vi "process.vi"() -> ()   [LabVIEW 2012]
uses:
  <vilib>/vision/Image Controls.llb/IMAQ Image.ctl
  <vilib>/vision/NI_Vision_Development_Module.lvlib
panel:
  out "targetCount":i32
  in  "Save":bool
  out "imageCount":i32
  in  "Existing Target":bool
  out "Identified Targets":T2(array[cluster]) {"Orientation" items=["North", "North-East", "East", "South-East", "South", "South-West", "West", "North-West"]; "Cluster"."Longitude" format="%#_10g"; "Cluster"."Latitude" format="%#_10g"}
  out "data":string
  out "state":i32
  in  "New Target Button":bool
  in  "currentImage":i32
  out "Image Out":T1(plugin-control)
  out "reloadImage":refnum<user-event>
  in  "prevbutton":bool
  in  "nextButton":bool
  in  "stop":bool
  out "Image Count":i32
  out "Available Images":i32[](array[numeric])
  # "of"
  # "of"
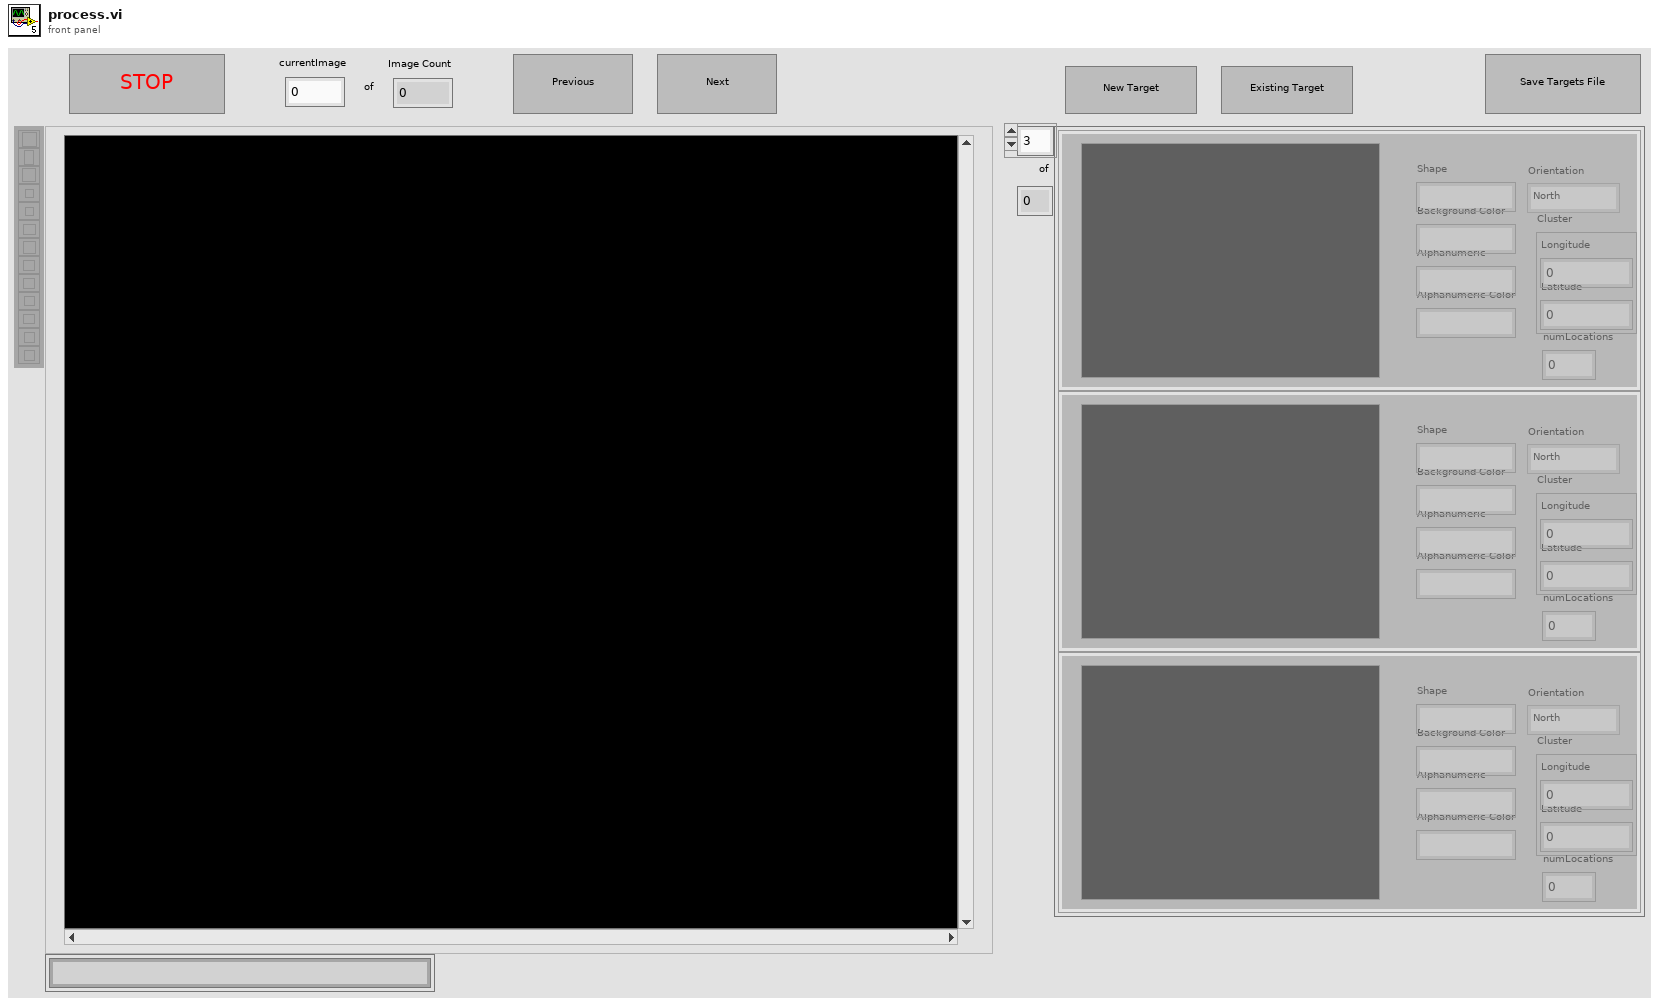
[diagram p1: front panel]
types:
  T1 = typedef "IMAQ Image.ctl" = refnum<image>
  T2 = cluster{"Image Out":T1, "Shape":string, "Background Color":string, "Alphanumeric":string, "Alphanumeric Color":string, "Cluster":cluster{"Longitude":dbl, "Latitude":dbl}, "Orientation":u16, "numLocations":i32}[]
  T3 = cluster{"Global Rectangle":i32[], "Contours":cluster{"Contour Type":u32, "ROI Type":u32, "Points":i32[]}[]}
  T4 = enum16{"open", "replace", "create", "open or create", "replace or create", "replace or create with confirmation"}
  T5 = cluster{"Shift":bool, "Ctrl":bool, "Alt":bool, "Cmd":bool, "Opt":bool}
  T6 = typedef "Image Type" = u32
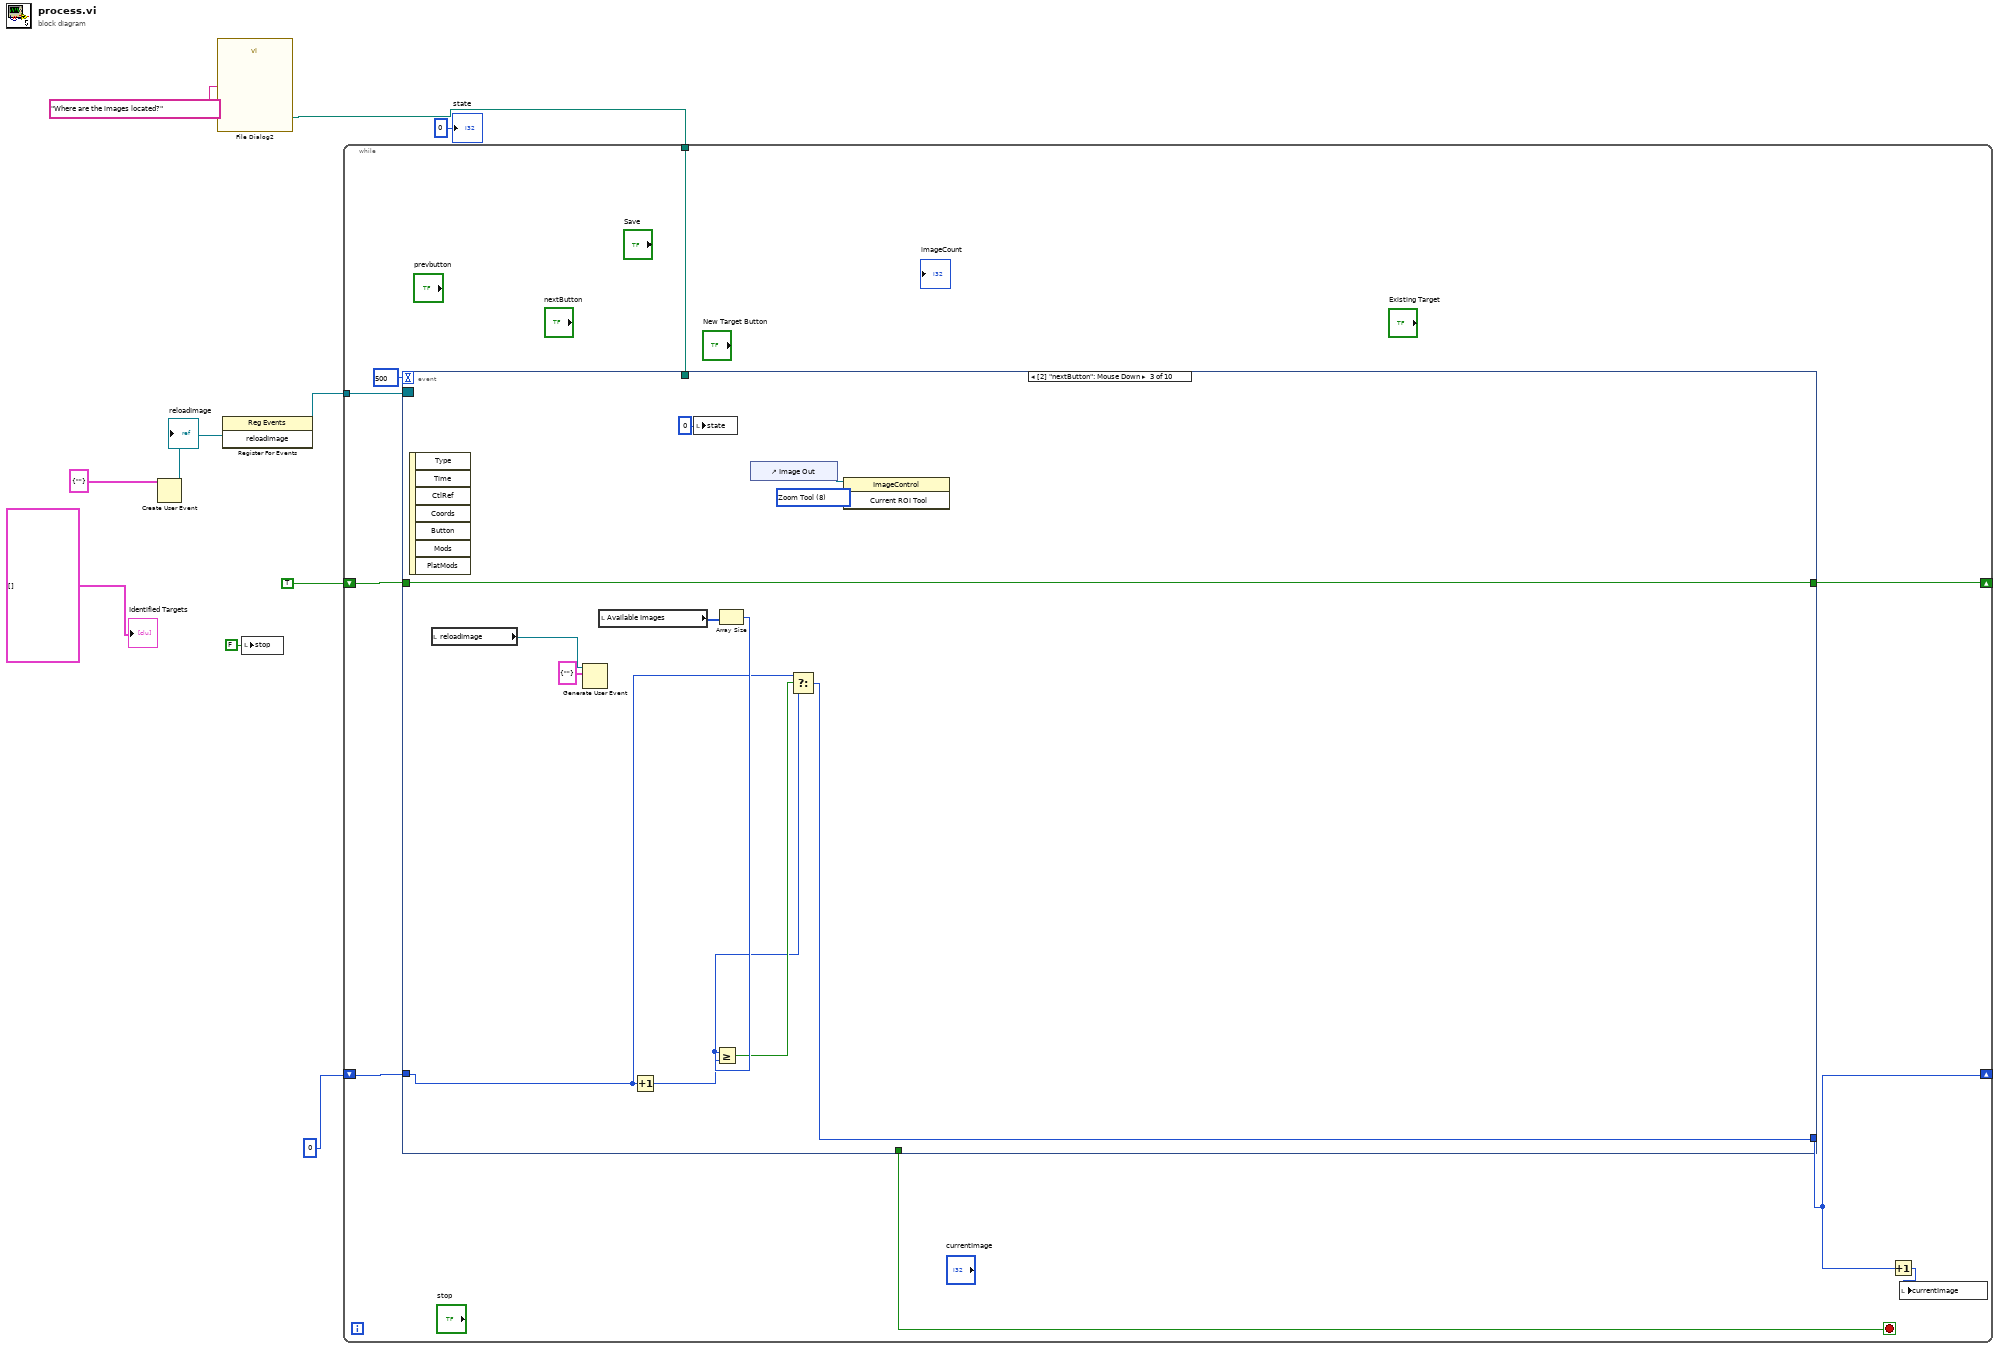
[diagram p0: block diagram]
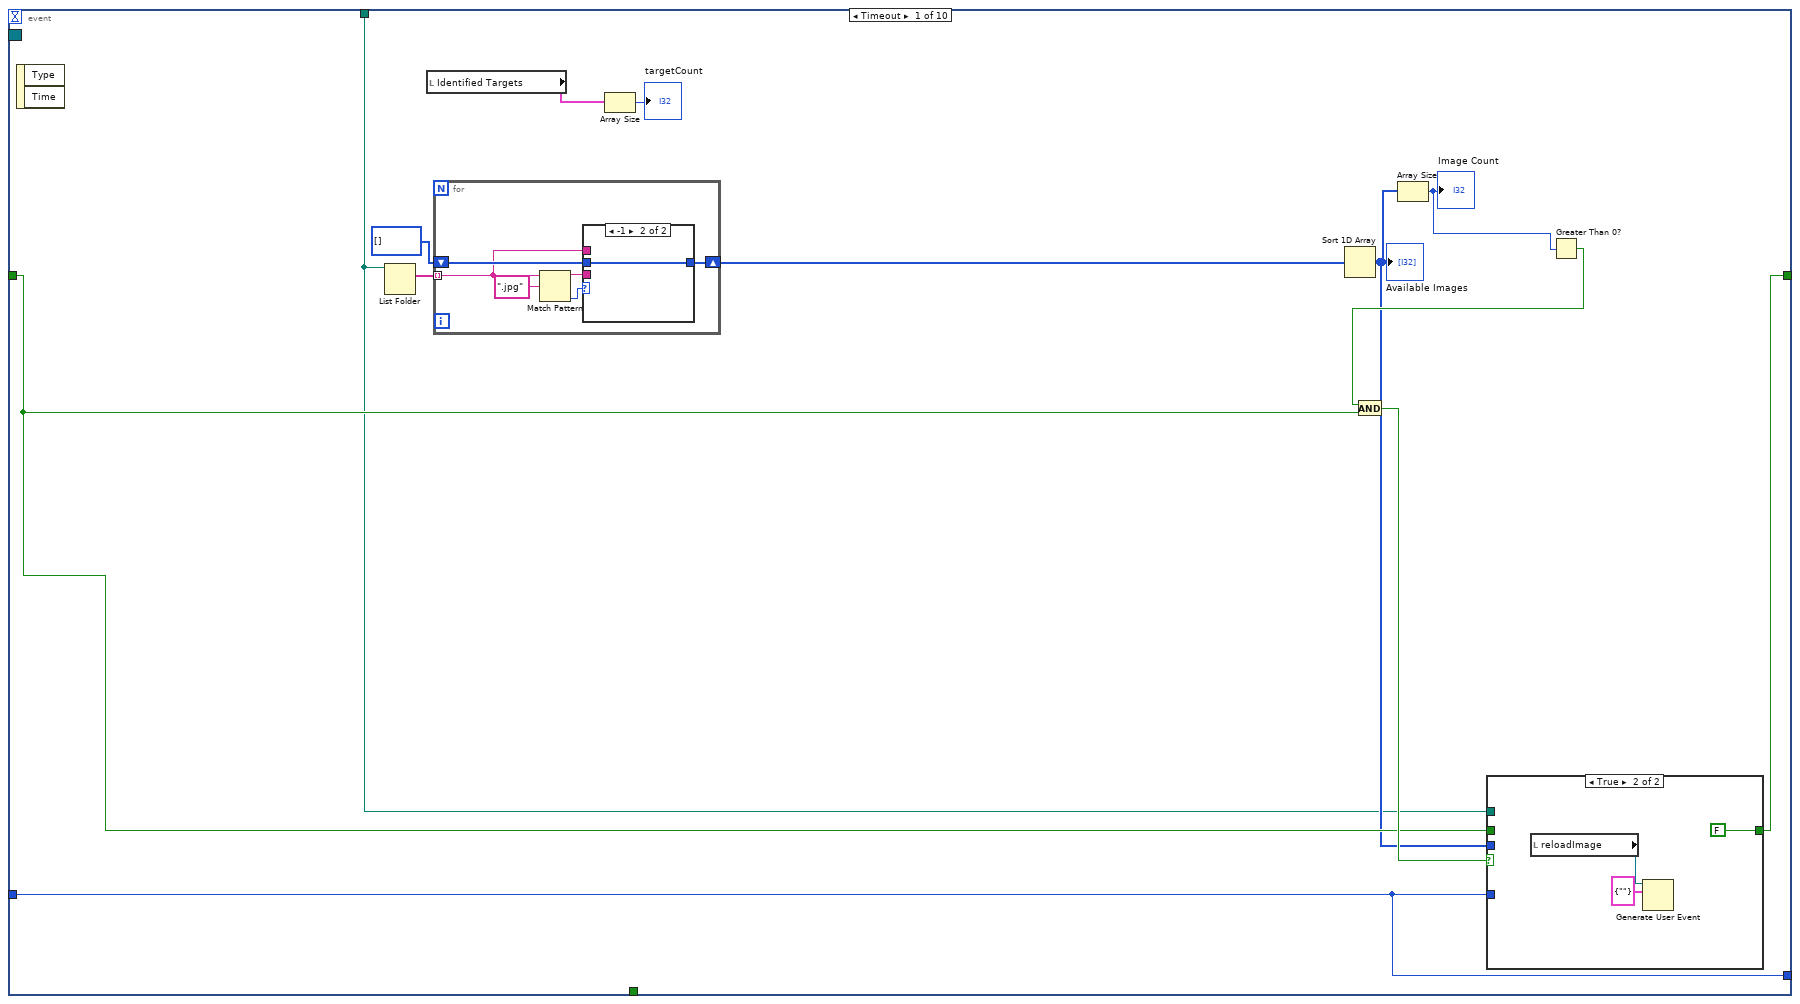
[diagram p2: hidden frame]
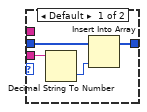
[diagram p4: hidden frame]
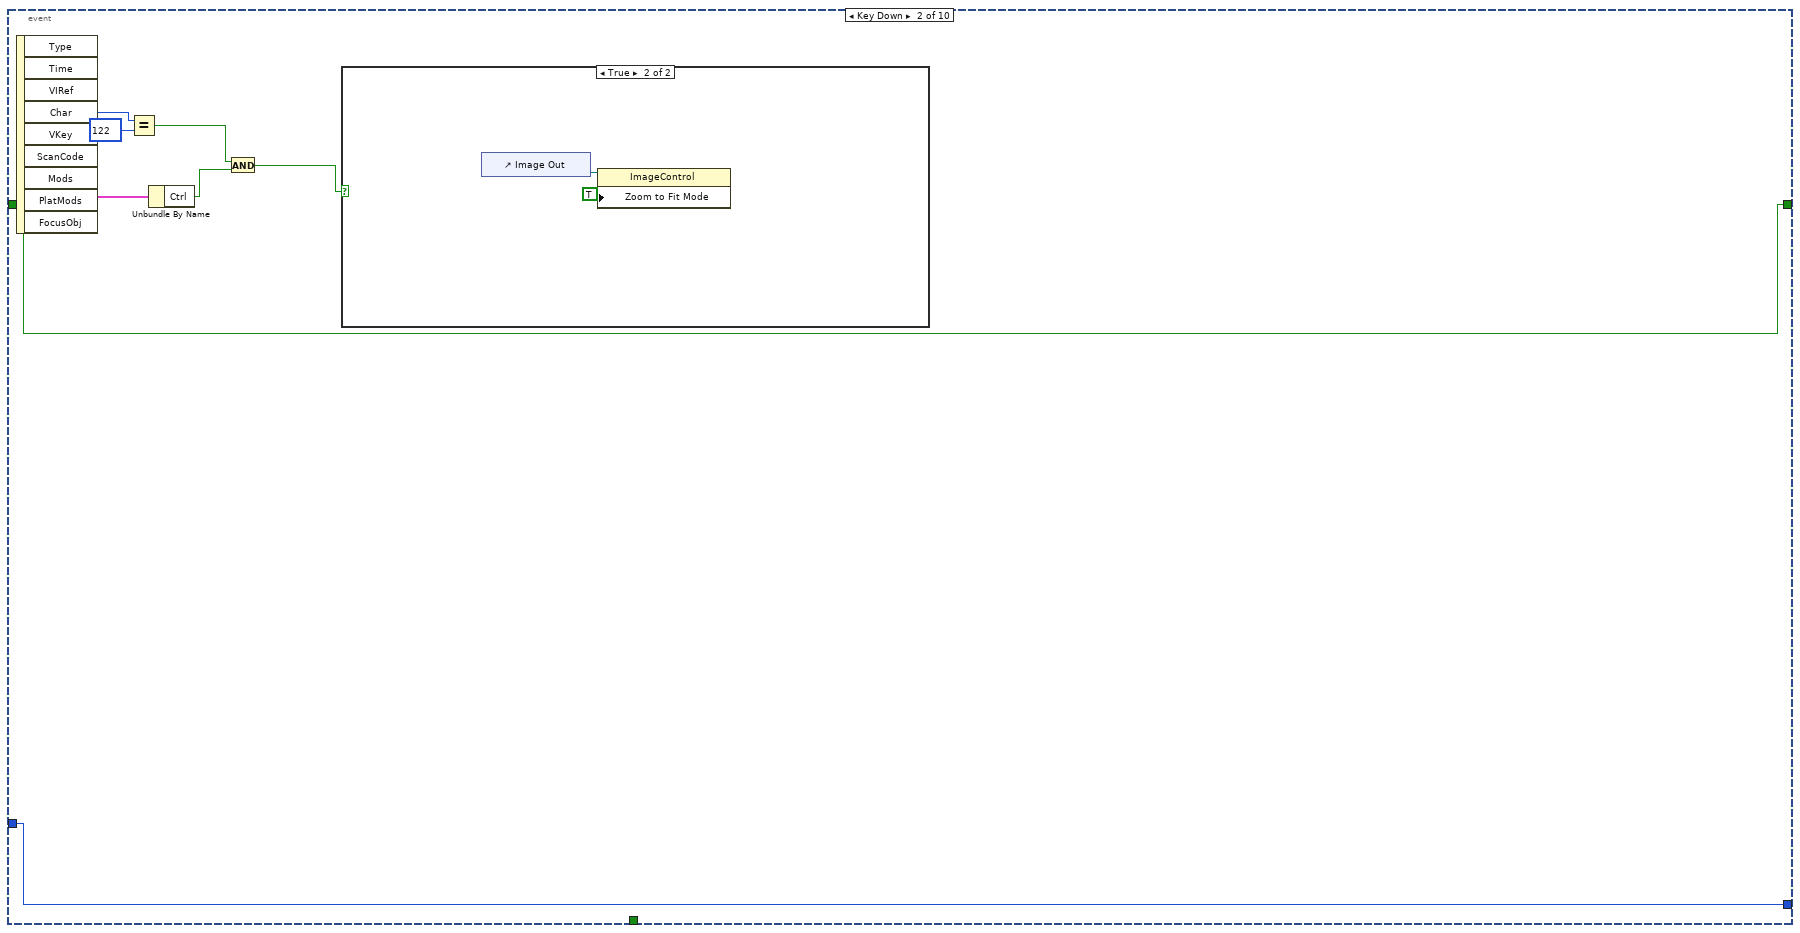
[diagram p5: hidden frame]
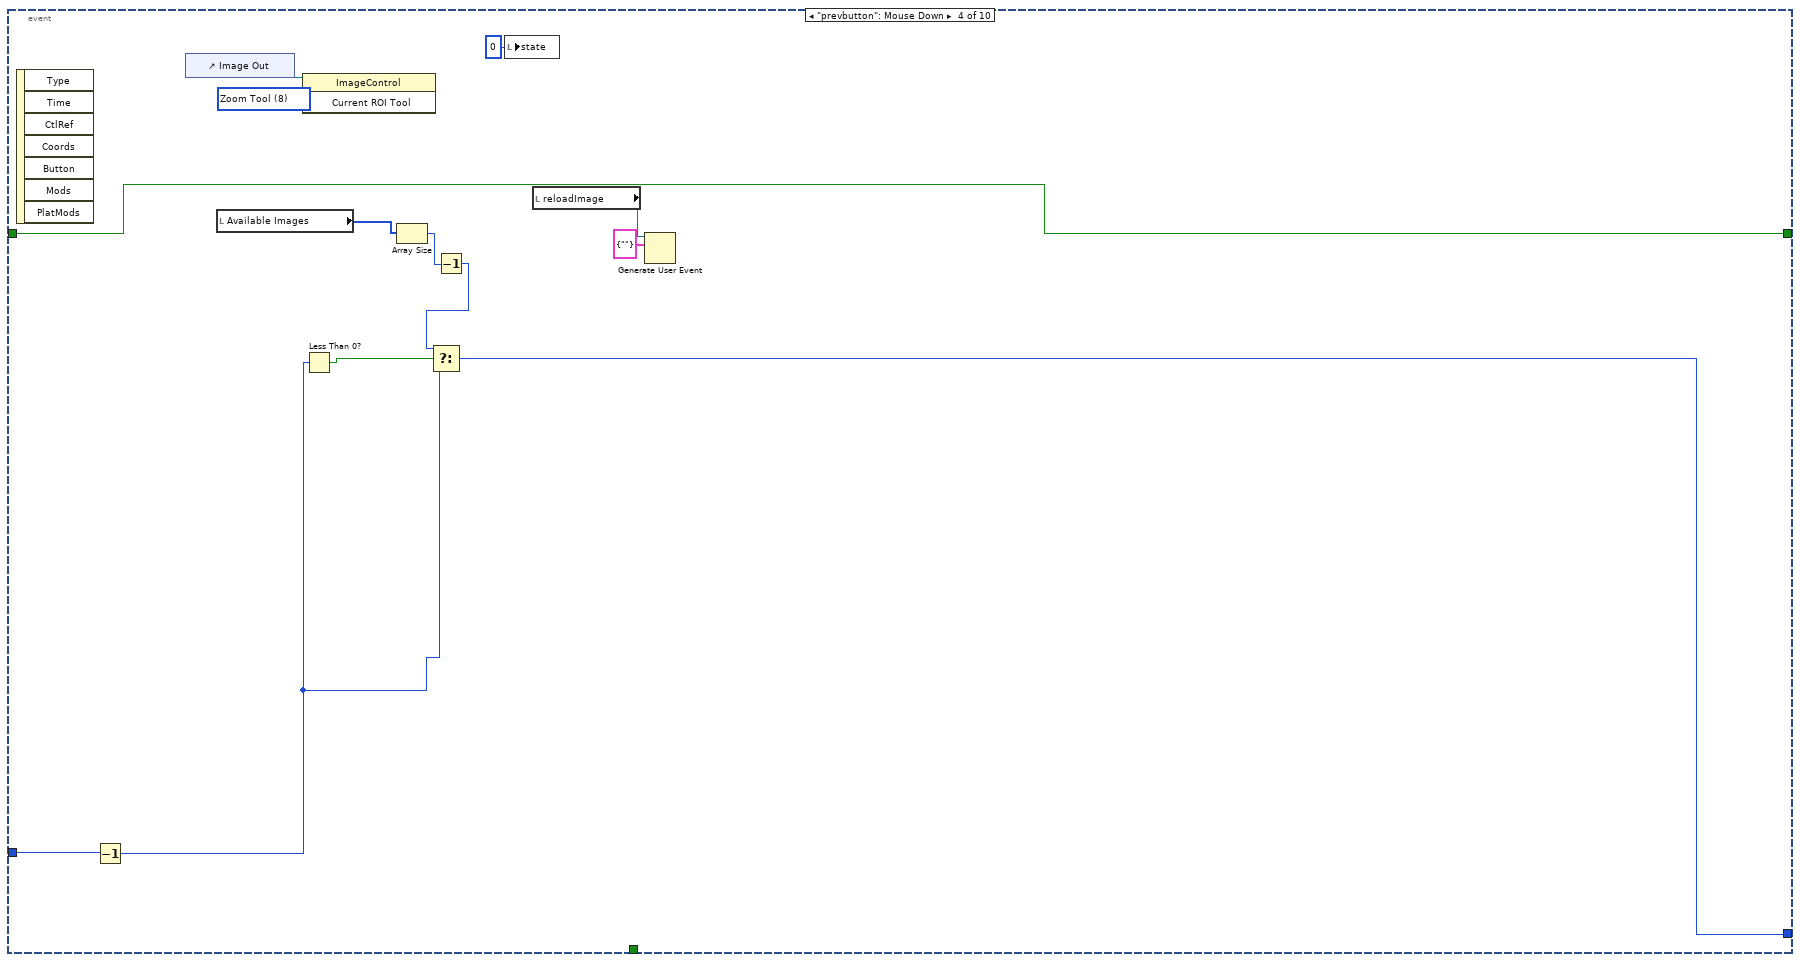
[diagram p7: hidden frame]
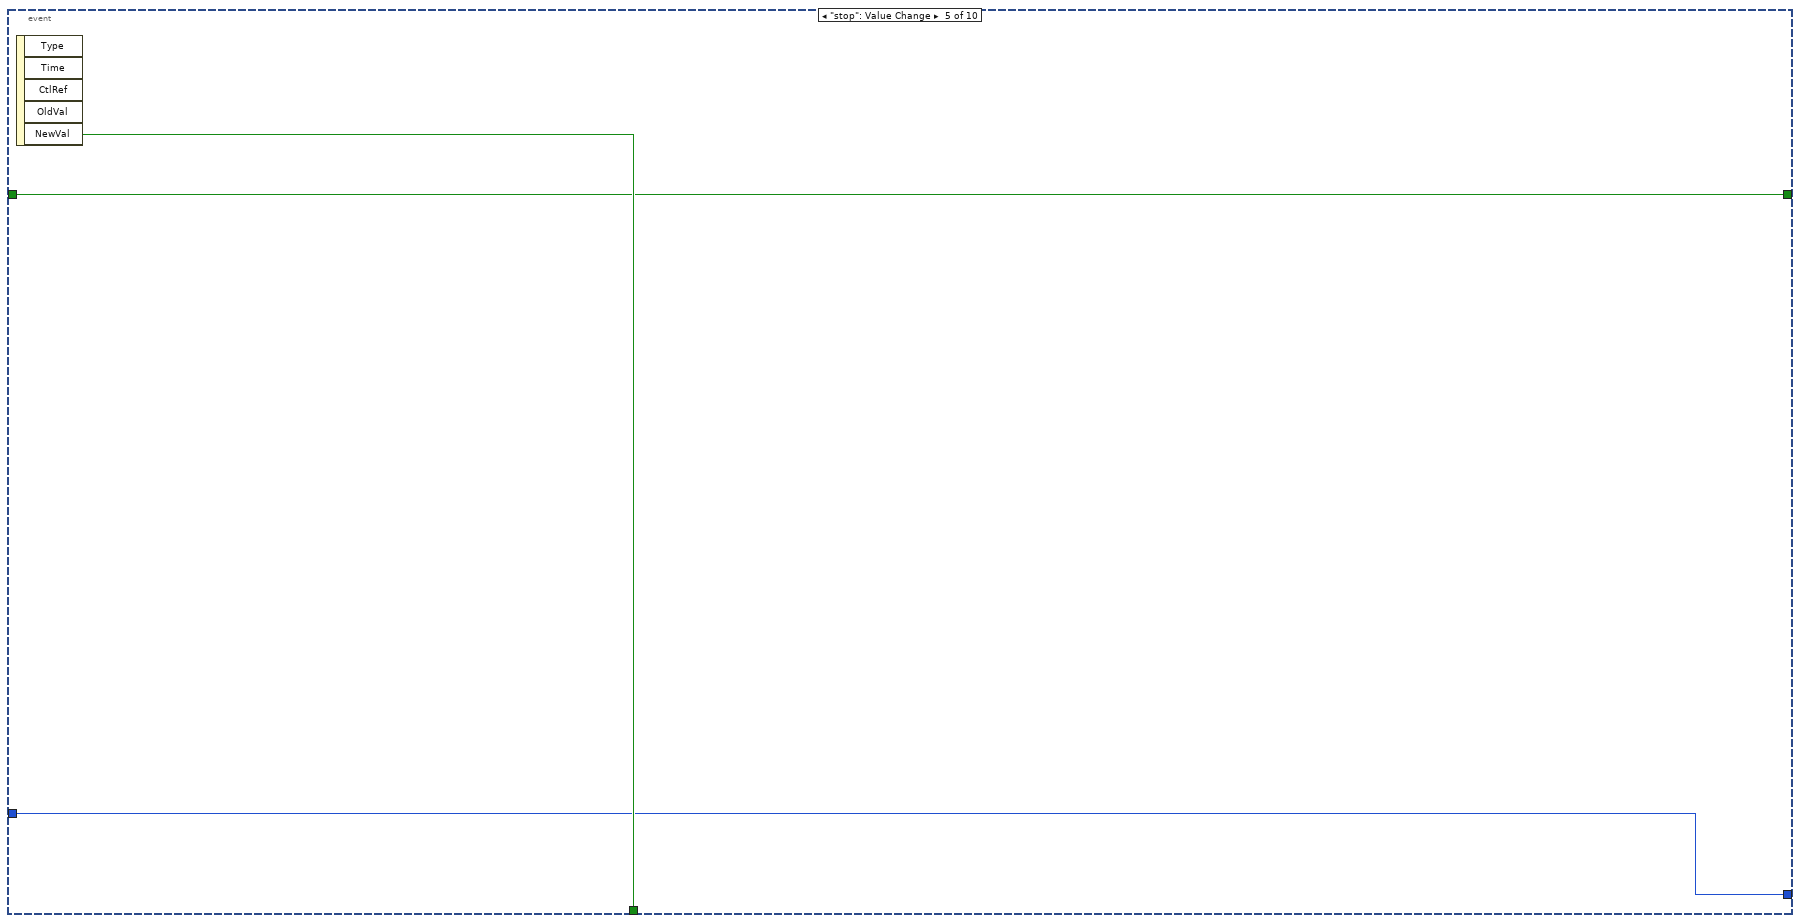
[diagram p8: hidden frame]
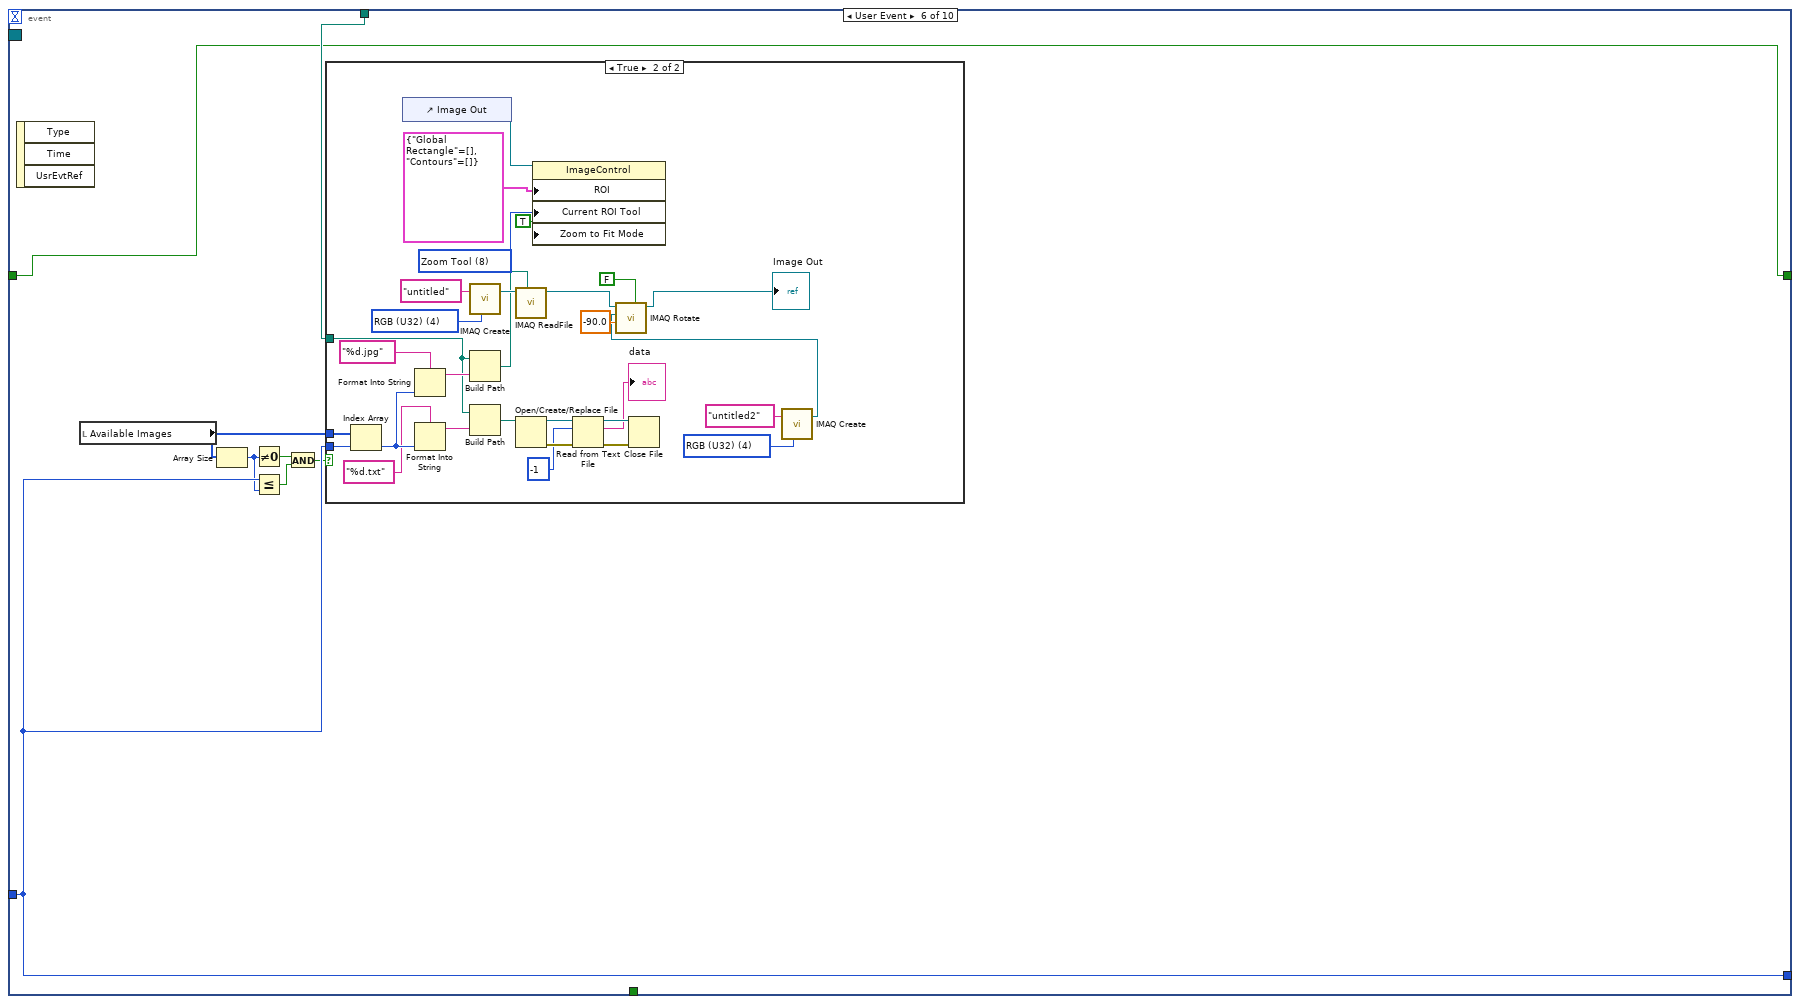
[diagram p9: hidden frame]
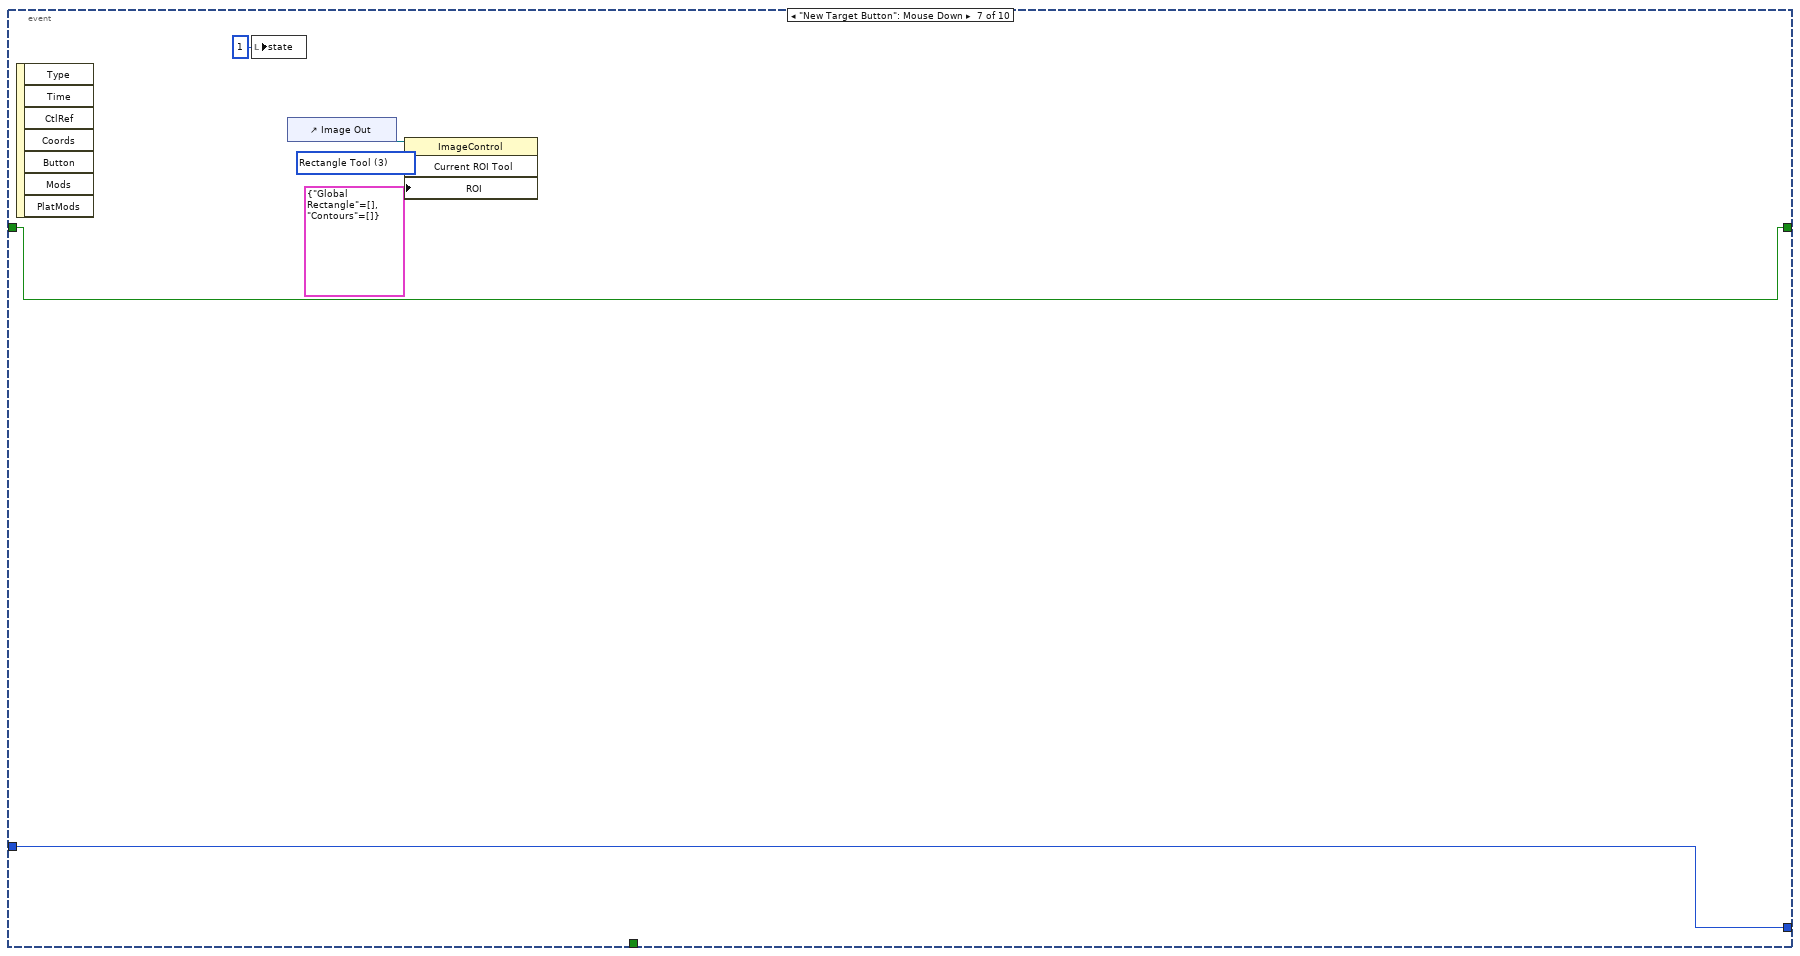
[diagram p11: hidden frame]
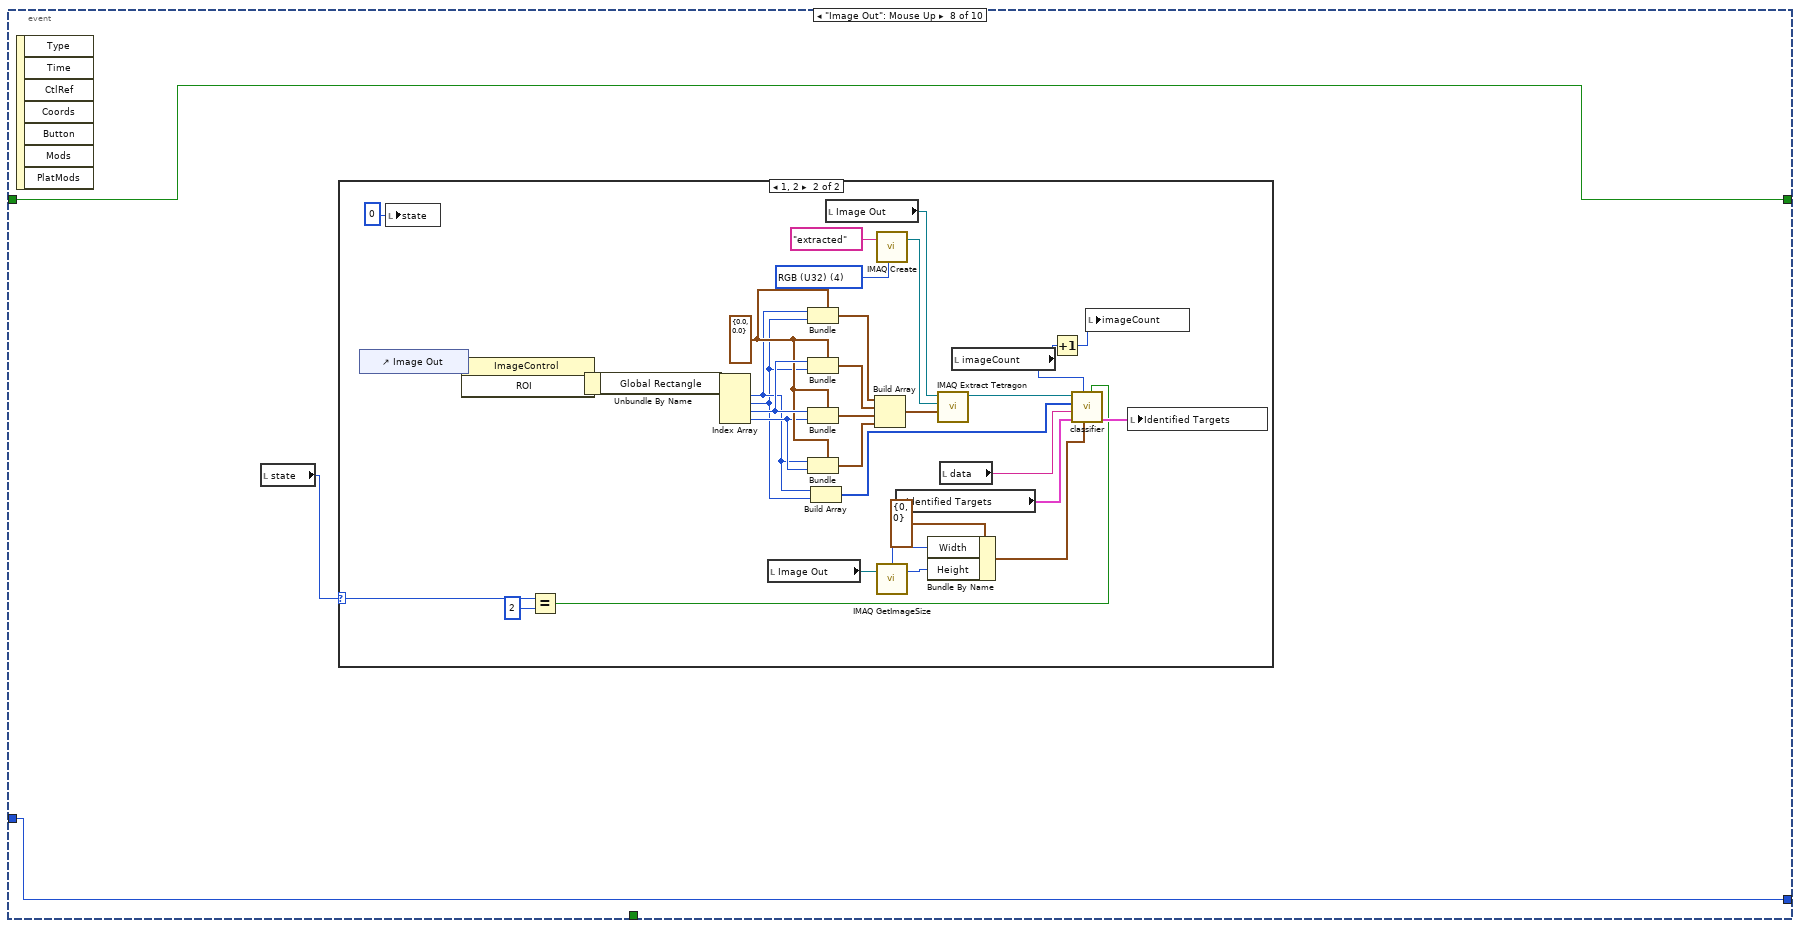
[diagram p12: hidden frame]
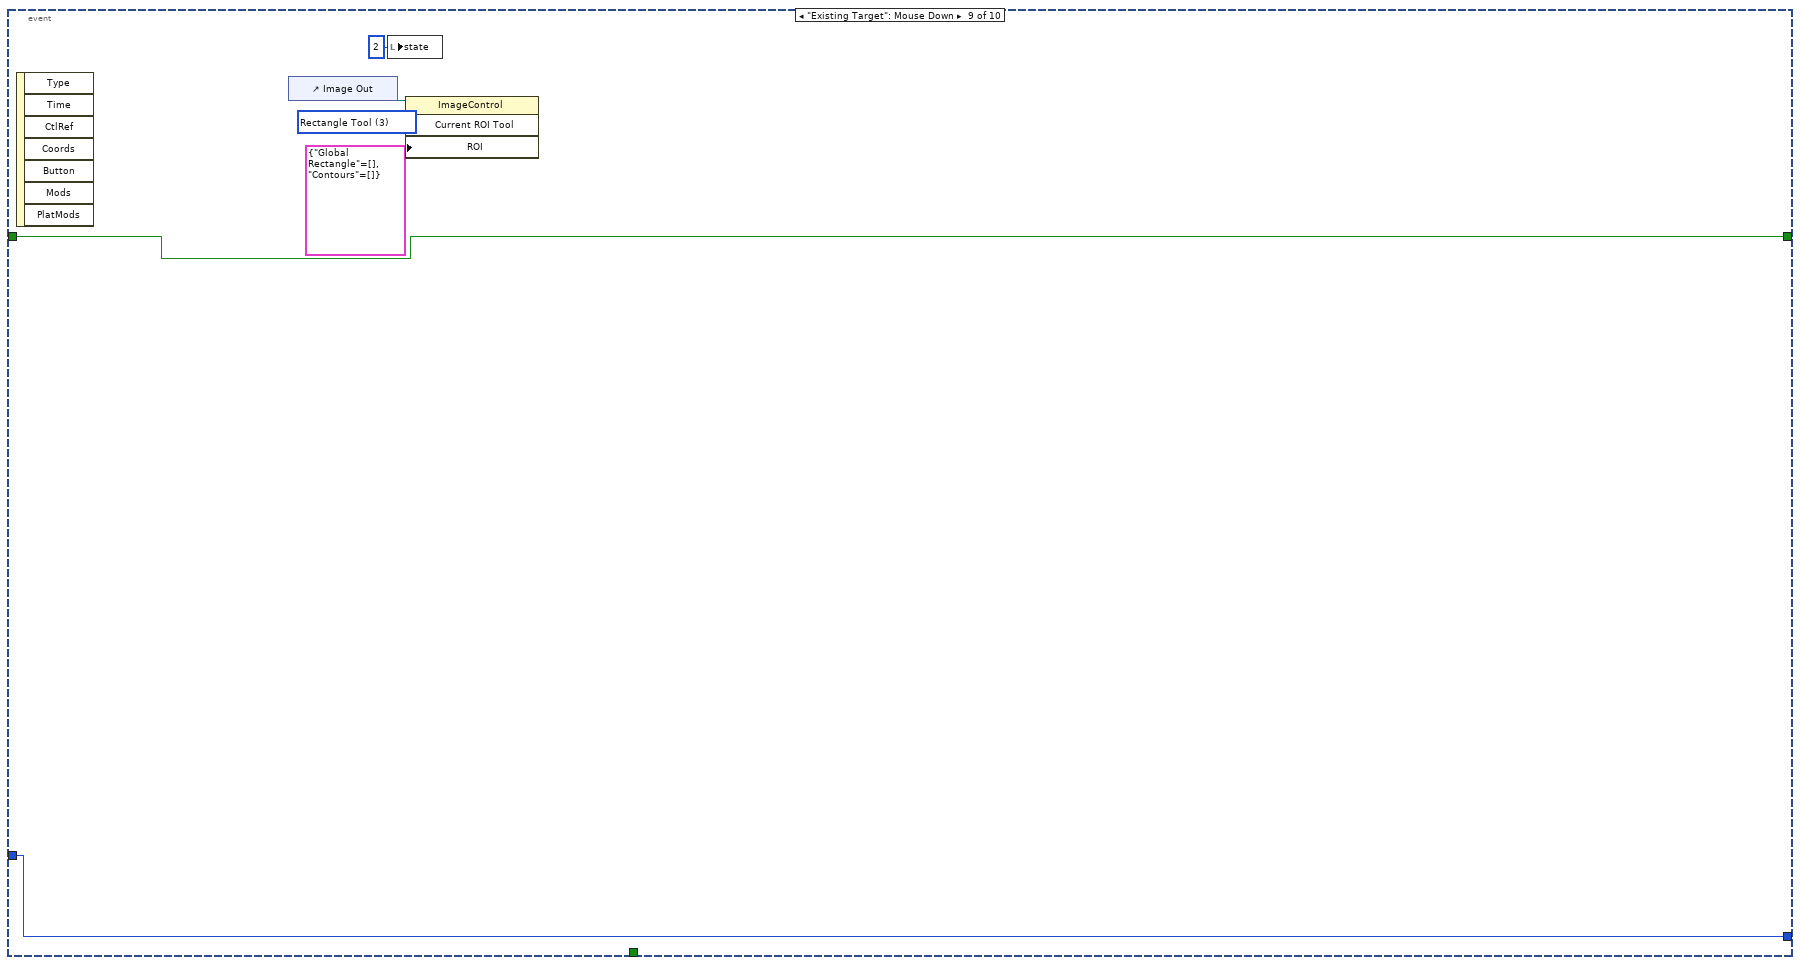
[diagram p14: hidden frame]
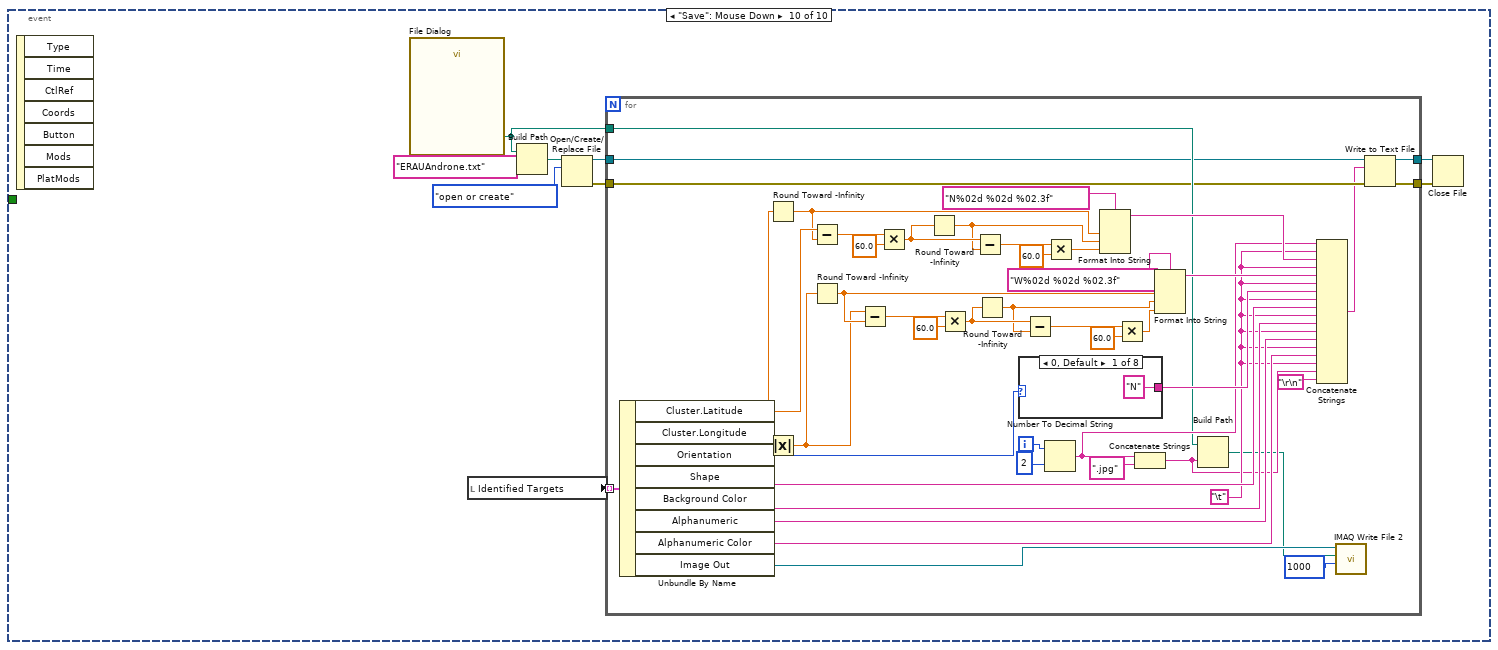
[diagram p15: hidden frame]
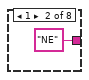
[diagram p16: hidden frame]
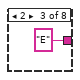
[diagram p17: hidden frame]
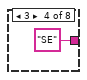
[diagram p18: hidden frame]
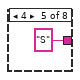
[diagram p19: hidden frame]
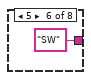
[diagram p20: hidden frame]
diagram:
  n1 = Create User Event(user event datatype=cluster{"stringy":string} {"stringy"=""} ("reloadImage")) -> (user event=w7:refnum<user-event>)  [unwired: 1 in, 1 out]
  "reloadImage" <- w7
  n2 = call "File Dialog2"("prompt"="Where are the images located?") -> ("selected path"=w3:path)  [unwired: 11 in, 3 out]
  n3 = register-events(w7) -> (reference out=w6:refnum<event-registration>)  [unwired: 2 in, 1 out]
  n4 = local write "stop"(FALSE ("stop")) -> ()
  n5 = while {
    shift-right: [w16] -> _
    shift-left: TRUE -> [w17]
    shift-right: [w14] -> _
    shift-left: 0 -> [w15]
    tunnel: w6 -> [w13]
    tunnel: w3 -> [w12]
    stop <- w18 stop-if-true
    n6 = event shown="[2] \"nextButton\": Mouse Down" {
      selector: w13 -> [_ _ _ _ _ _ _ _ _ _]
      dyn-events: _ -> [_ _ _ _ _ _ _ _ _ _]
      timeout: 500 -> [_ _ _ _ _ _ _ _ _ _]
      tunnel: [_ _ _ _ w85 _ _ _ _ _] -> w18
      tunnel: w17 -> [w25 w48 w69 w73 w83 w86 w126 w132 w166 _]
      tunnel: [w26 w48 w69 w73 w83 w86 w126 w132 w166 _] -> w16
      tunnel: w15 -> [w23 w49 w61 w82 w84 w92 w125 w131 w167 _]
      tunnel: [w23 w49 w62 w79 w84 w92 w125 w131 w167 _] -> w14
      tunnel: w12 -> [w22 _ _ _ _ w87 _ _ _ _]
      event Timeout {
        n7 = event-data() -> ()  [unwired: 1 in, 2 out]
        n8 = List Folder(path=w22) -> (filenames=w32:string[])  [unwired: 3 in, 3 out]
        n9 = local read "Identified Targets"() -> (w21:T2)
        n10 = for {
          tunnel: w32 -> [w39] mode=indexing
          shift-right: [w38] -> w30
          shift-left: i32[] [] -> [w40]
          n11 = Match Pattern(string=w39, regular expression=".jpg") -> (before substring=w37:string, offset past match=w41:i32)  [unwired: 1 in, 2 out]
          n12 = case shown="-1" w41 {
            tunnel: w40 -> [w46 w47]
            tunnel: w39 -> [_ _]
            tunnel: [w45 w47] -> w38
            tunnel: w37 -> [w44 _]
            frame Default {
              n13 = Decimal String To Number(string=w44) -> (number=w43:i32)  [unwired: 2 in, 1 out]
              n14 = Insert Into Array(array=w46, new element=w43) -> (w45:i32[])  [unwired: 1 in]
            }
            frame -1 {
            }
          }
        }
        n15 = Array Size(array=w21) -> (size(s)=→"targetCount":i32)
        n16 = Sort 1D Array(array=w30) -> (sorted array=w24:i32[])
        "Available Images" <- w24
        n17 = Array Size(array=w24) -> (size(s)=w28:i32)
        "Image Count" <- w28
        n18 = Greater Than 0?(x=w28) -> (x > 0?=w27:bool)
        n19 = And(x=w27, y=w25) -> (x .and. y?=w29:bool)
        n20 = case shown="True" w29 {
          tunnel: [w33 FALSE] -> w26
          tunnel: w25 -> [w33 _]
          tunnel: w24 -> [_ _]
          tunnel: w23 -> [_ _]
          tunnel: w22 -> [_ _]
          frame False {
          }
          frame True {
            n21 = local read "reloadImage"() -> (w35:refnum<user-event>)
            n22 = Generate User Event(user event=w35, event data cluster=cluster{"stringy":string} {"stringy"=""} ("event data")) -> ()  [unwired: 1 in, 2 out]
          }
        }
      }
      event Key Down {
        n23 = event-data() -> ("Char"=w54:i16, "PlatMods"=w55:T5)  [unwired: 1 in, 7 out]
        n24 = Equal?(x=w54, y=i16 122) -> (x = y?=w51:bool)
        n25 = Unbundle By Name(w55) -> ("Ctrl"=w52:bool)
        n26 = And(x=w51, y=w52) -> (x .and. y?=w50:bool)
        n27 = case shown="True" w50 {
          frame False {
          }
          frame True {
            n28 = control-ref of="Image Out"() -> (w57:refnum<vi>)
            n29 = property class="ImageControl"(reference=w57, "Zoom to Fit Mode"=TRUE) -> ()  [unwired: 1 in, 2 out]
          }
        }
      }
      event "nextButton": Mouse Down {
        w58 = u32 8 items=["Zoom Tool"=8, "Selection Tool"=0, "Pan Tool"=9, "Point Tool"=1, "Line Tool"=2, "Rectangle Tool"=3, "Rotated Rectangle Tool"=12, "Polyline Tool"=10, "Polygon Tool"=5, "Freehand Tool"=11, "Closed Freehand Tool"=6, "Ellipse Tool"=4, "Annulus Tool"=7] ("Current ROI Tool")
        n30 = event-data() -> ()  [unwired: 1 in, 7 out]
        n31 = local read "reloadImage"() -> (w68:refnum<user-event>)
        n32 = Generate User Event(user event=w68, event data cluster=cluster{"stringy":string} {"stringy"=""} ("event data")) -> ()  [unwired: 1 in, 2 out]
        n33 = local read "Available Images"() -> (w66:i32[])
        n34 = Increment(x=w61) -> (x+1=w63:i32)
        n35 = local write "state"(0 ("state")) -> ()
        n36 = Array Size(array=w66) -> (size(s)=w65:i32)
        n37 = Greater Or Equal?(x=w63, y=w65) -> (x >= y?=w64:bool)
        n38 = control-ref of="Image Out"() -> (w59:refnum<vi>)
        n39 = Select(t=w61, s=w64, f=w63) -> (s? t:f=w62:i32)
        n40 = property class="ImageControl"(reference=w59, "Current ROI Tool"=w58) -> ()  [unwired: 1 in, 2 out]
      }
      event "prevbutton": Mouse Down {
        w70 = u32 8 items=["Zoom Tool"=8, "Selection Tool"=0, "Pan Tool"=9, "Point Tool"=1, "Line Tool"=2, "Rectangle Tool"=3, "Rotated Rectangle Tool"=12, "Polyline Tool"=10, "Polygon Tool"=5, "Freehand Tool"=11, "Closed Freehand Tool"=6, "Ellipse Tool"=4, "Annulus Tool"=7] ("Current ROI Tool")
        n41 = event-data() -> ()  [unwired: 1 in, 7 out]
        n42 = Decrement(x=w82) -> (x-1=w80:i32)
        n43 = control-ref of="Image Out"() -> (w71:refnum<vi>)
        n44 = local read "Available Images"() -> (w78:i32[])
        n45 = property class="ImageControl"(reference=w71, "Current ROI Tool"=w70) -> ()  [unwired: 1 in, 2 out]
        n46 = Less Than 0?(x=w80) -> (x < 0?=w81:bool)
        n47 = Array Size(array=w78) -> (size(s)=w77:i32)
        n48 = Decrement(x=w77) -> (x-1=w76:i32)
        n49 = Select(t=w76, s=w81, f=w80) -> (s? t:f=w79:i32)
        n50 = local write "state"(0 ("state")) -> ()
        n51 = local read "reloadImage"() -> (w75:refnum<user-event>)
        n52 = Generate User Event(user event=w75, event data cluster=cluster{"stringy":string} {"stringy"=""} ("event data")) -> ()  [unwired: 1 in, 2 out]
      }
      event "stop": Value Change {
        n53 = event-data() -> ("NewVal"=w85:bool)  [unwired: 1 in, 4 out]
      }
      event User Event {
        n54 = event-data() -> ()  [unwired: 1 in, 3 out]
        n55 = local read "Available Images"() -> (w93:i32[])
        n56 = Array Size(array=w93) -> (size(s)=w91:i32)
        n57 = Not Equal To 0?(x=w91) -> (x != 0?=w90:bool)
        n58 = Less Or Equal?(x=w92, y=w91) -> (x <= y?=w89:bool)
        n59 = And(x=w90, y=w89) -> (x .and. y?=w88:bool)
        n60 = case shown="True" w88 {
          tunnel: w92 -> [_ w117]
          tunnel: w93 -> [_ w116]
          tunnel: w87 -> [_ w111]
          frame False {
          }
          frame True {
            w99 = T6 4 items=["Grayscale (U8)", "Grayscale (I16)", "Grayscale (SGL)", "Complex (CSG)", "RGB (U32)", "HSL (U32)", "RGB (U64)", "Grayscale (U16)"] ("Image Type")
            w102 = u32 8 items=["Zoom Tool"=8, "Selection Tool"=0, "Pan Tool"=9, "Point Tool"=1, "Line Tool"=2, "Rectangle Tool"=3, "Rotated Rectangle Tool"=12, "Polyline Tool"=10, "Polygon Tool"=5, "Freehand Tool"=11, "Closed Freehand Tool"=6, "Ellipse Tool"=4, "Annulus Tool"=7] ("Current ROI Tool")
            w118 = T6 4 items=["Grayscale (U8)", "Grayscale (I16)", "Grayscale (SGL)", "Complex (CSG)", "RGB (U32)", "HSL (U32)", "RGB (U64)", "Grayscale (U16)"] ("Image Type")
            n61 = Index Array(array=w116, index=w117) -> (element=w113:i32)
            n62 = control-ref of="Image Out"() -> (w115:refnum<vi>)
            n63 = Format Into String(format string="%d.jpg", w113) -> (resulting string=w120:string)  [unwired: 2 in, 1 out]
            n64 = Format Into String(format string="%d.txt", w113) -> (resulting string=w110:string)  [unwired: 2 in, 1 out]
            n65 = call "IMAQ Create"("Image Name"="untitled", "Image Type"=w118) -> ("New Image"=w123:T1)  [unwired: 3 in, 1 out]
            n66 = Build Path(base path=w111, name or relative path=w120) -> (appended path=w119:path)
            n67 = Build Path(base path=w111, name or relative path=w110) -> (appended path=w109:path)
            n68 = call "IMAQ ReadFile"("File Path"=w119, "Image"=w123) -> ("Image Out"=w95:T1)  [unwired: 5 in, 4 out]
            n69 = Open/Create/Replace File(file path (use dialog)=w109) -> (refnum out=w108:refnum<file>, error out=w107:errorcluster)  [unwired: 5 in, 1 out]
            n70 = property class="ImageControl"(reference=w115, "ROI"=T3 {"Global Rectangle"=[], "Contours"=[]}, "Current ROI Tool"=w102, "Zoom to Fit Mode"=TRUE) -> ()  [unwired: 1 in, 2 out]
            n71 = Read from Text File(file (use dialog)=w108, count=-1, error in=w107) -> (refnum out=w105:refnum<file>, text=→"data":string, error out=w104:errorcluster)  [unwired: 1 in, 1 out]
            n72 = Close File(refnum=w105, error in=w104) -> ()  [unwired: 2 out]
            n73 = call "IMAQ Create"("Image Name"="untitled2", "Image Type"=w99) -> ("New Image"=w97:T1)  [unwired: 3 in, 1 out]
            n74 = call "IMAQ Rotate"("Maintain Size"=FALSE, "Angle (degrees)"=sgl -90.0, "Image Dst"=w97, "Image Src"=w95) -> ("Image Dst Out"=→"Image Out":T1)  [unwired: 6 in, 1 out]
          }
        }
      }
      event "New Target Button": Mouse Down {
        w128 = u32 3 items=["Zoom Tool"=8, "Selection Tool"=0, "Pan Tool"=9, "Point Tool"=1, "Line Tool"=2, "Rectangle Tool"=3, "Rotated Rectangle Tool"=12, "Polyline Tool"=10, "Polygon Tool"=5, "Freehand Tool"=11, "Closed Freehand Tool"=6, "Ellipse Tool"=4, "Annulus Tool"=7] ("Current ROI Tool")
        n75 = event-data() -> ()  [unwired: 1 in, 7 out]
        n76 = local write "state"(1 ("state")) -> ()
        n77 = control-ref of="Image Out"() -> (w129:refnum<vi>)
        n78 = property class="ImageControl"(reference=w129, "Current ROI Tool"=w128, "ROI"=T3 {"Global Rectangle"=[], "Contours"=[]}) -> ()  [unwired: 1 in, 2 out]
      }
      event "Image Out": Mouse Up {
        n79 = event-data() -> ()  [unwired: 1 in, 7 out]
        n80 = local read "state"() -> (w130:i32)
        n81 = case shown="1, 2" w130 {
          selector: w130 -> [_ w137]
          frame Default {
          }
          frame 1, 2 {
            w155 = cluster{"x":sgl, "y":sgl} {"x"=0.0, "y"=0.0}
            w163 = T6 4 items=["Grayscale (U8)", "Grayscale (I16)", "Grayscale (SGL)", "Complex (CSG)", "RGB (U32)", "HSL (U32)", "RGB (U64)", "Grayscale (U16)"] ("Image Type")
            n82 = control-ref of="Image Out"() -> (w165:refnum<vi>)
            n83 = local write "state"(0 ("state")) -> ()
            n84 = property class="ImageControl"(reference=w165) -> ("ROI"=w162:T3)  [unwired: 1 in, 2 out]
            n85 = Equal?(x=w137, y=2) -> (x = y?=w135:bool)
            n86 = Unbundle By Name(w162) -> ("Global Rectangle"=w161:i32[])
            n87 = Index Array(array=w161) -> (element #1=w149:i32, element #2=w148:i32, element #3=w156:i32, element #4=w154:i32)  [unwired: 4 in]
            n88 = local read "Image Out"() -> (w142:T1)
            n89 = Bundle(cluster=w155, "x"=w149, "y"=w148) -> (w158:cluster{"x":sgl, "y":sgl})
            n90 = Bundle(cluster=w155, "x"=w156, "y"=w148) -> (w153:cluster{"x":sgl, "y":sgl})
            n91 = Bundle(cluster=w155, "x"=w156, "y"=w154) -> (w152:cluster{"x":sgl, "y":sgl})
            n92 = Bundle(cluster=w155, "x"=w149, "y"=w154) -> (w151:cluster{"x":sgl, "y":sgl})
            n93 = Build Array(w149, w148) -> (w147:i32[])
            n94 = local read "Image Out"() -> (w160:T1)
            n95 = Build Array(w158, w153, w152, w151) -> (w157:cluster{"x":sgl, "y":sgl}[])
            n96 = call "IMAQ Create"("Image Name"="extracted", "Image Type"=w163) -> ("New Image"=w159:T1)  [unwired: 3 in, 1 out]
            n97 = call "IMAQ GetImageSize"("Image"=w142) -> ("Y Resolution"=w140:i32, "X Resolution"=w139:i32)  [unwired: 3 in, 1 out]
            n98 = local read "Identified Targets"() -> (w144:T2)
            n99 = Bundle By Name(cluster=cluster{"Width":u32, "Height":u32} {"Width"=0, "Height"=0} ("Displayed Image:Size:All Elements"), "Width"=w139, "Height"=w140) -> (w138:cluster{"Width":u32, "Height":u32})
            n100 = call-poly "IMAQ Extract Tetragon"("Tetragon"=w157, "Image Dst"=w159, "Image Src"=w160) -> ("Image Dst Out"=w150:T1)  [unwired: 7 in, 1 out]
            n101 = local read "data"() -> (w145:string)
            n102 = local read "imageCount"() -> (w134:i32)
            n103 = Increment(x=w134) -> (x+1=w133:i32)
            n104 = call "classifier.vi"("existingTarget"=w135, "ImageSize"=w138, "targetCount"=w134, "input array"=w144, "data"=w145, "InitialValues"=w147, "Image In"=w150) -> ("output array"=w143:T2)  [unwired: 4 in]
            n105 = local write "imageCount"(w133) -> ()
            n106 = local write "Identified Targets"(w143) -> ()
          }
        }
      }
      event "Existing Target": Mouse Down {
        w170 = u32 3 items=["Zoom Tool"=8, "Selection Tool"=0, "Pan Tool"=9, "Point Tool"=1, "Line Tool"=2, "Rectangle Tool"=3, "Rotated Rectangle Tool"=12, "Polyline Tool"=10, "Polygon Tool"=5, "Freehand Tool"=11, "Closed Freehand Tool"=6, "Ellipse Tool"=4, "Annulus Tool"=7] ("Current ROI Tool")
        n107 = event-data() -> ()  [unwired: 1 in, 7 out]
        n108 = control-ref of="Image Out"() -> (w171:refnum<vi>)
        n109 = local write "state"(2 ("state")) -> ()
        n110 = property class="ImageControl"(reference=w171, "Current ROI Tool"=w170, "ROI"=T3 {"Global Rectangle"=[], "Contours"=[]}) -> ()  [unwired: 1 in, 2 out]
      }
      event "Save": Mouse Down {
        n111 = event-data() -> ()  [unwired: 1 in, 7 out]
        n112 = call "File Dialog"() -> ("selected path"=w178:path)  [unwired: 12 in, 3 out]
        n113 = local read "Identified Targets"() -> (w180:T2)
        n114 = Build Path(base path=w178, name or relative path="ERAUAndrone.txt") -> (appended path=w177:path)
        n115 = Open/Create/Replace File(file path (use dialog)=w177, operation (0:open)=T4."open or create") -> (refnum out=w175:refnum<file>, error out=w174:errorcluster)  [unwired: 4 in, 1 out]
        n116 = for {
          tunnel: w180 -> [w224] mode=indexing
          tunnel: w178 -> [w191]
          tunnel: w175 -> [w185]
          tunnel: w174 -> [w184]
          tunnel: [w182] -> w173
          tunnel: [w181] -> w172
          i -> [w226]
          w192 = "\t"
          n117 = Unbundle By Name(w224) -> ("Cluster.Latitude"=w222:dbl, "Cluster.Longitude"=w208:dbl, "Orientation"=w200:u16, "Shape"=w198:string, "Background Color"=w197:string, "Alphanumeric"=w196:string, "Alphanumeric Color"=w195:string, "Image Out"=w189:T1)
          n118 = Round Toward -Infinity(1:w222) -> (0:w221:dbl)
          n119 = Absolute Value(x=w208) -> (abs(x)=w201:dbl)
          n120 = Subtract(x=w222, y=w221) -> (x-y=w218:dbl)
          n121 = Round Toward -Infinity(1:w201) -> (0:w210:dbl)
          n122 = Subtract(x=w201, y=w210) -> (x-y=w213:dbl)
          n123 = Multiply(x=w218, y=60.0) -> (x*y=w205:dbl)
          n124 = Round Toward -Infinity(1:w205) -> (0:w204:dbl)
          n125 = Multiply(x=w213, y=60.0) -> (x*y=w203:dbl)
          n126 = Subtract(x=w205, y=w204) -> (x-y=w217:dbl)
          n127 = Round Toward -Infinity(1:w203) -> (0:w202:dbl)
          n128 = case shown="0, Default" w200 {
            tunnel: ["N" "NE" "E" "SE" "S" "SW" "W" "NW"] -> w199
            frame 0, Default {
            }
            frame 1 {
            }
            frame 2 {
            }
            frame 3 {
            }
            frame 4 {
            }
            frame 5 {
            }
            frame 6 {
            }
            frame 7 {
            }
          }
          n129 = Subtract(x=w203, y=w202) -> (x-y=w214:dbl)
          n130 = Number To Decimal String(number=w226, width (-)=i16 2) -> (decimal integer string=w194:string)
          n131 = Multiply(x=w217, y=60.0) -> (x*y=w216:dbl)
          n132 = Format Into String(format string="N%02d %02d %02.3f", w221, w204, w216) -> (resulting string=w207:string)  [unwired: 2 in, 1 out]
          n133 = Multiply(x=w214, y=60.0) -> (x*y=w215:dbl)
          n134 = Concatenate Strings(w194, ".jpg" ("string")) -> (w190:string)
          n135 = Format Into String(format string="W%02d %02d %02.3f", w210, w202, w215) -> (resulting string=w206:string)  [unwired: 2 in, 1 out]
          n136 = Build Path(base path=w191, name or relative path=w190) -> (appended path=w188:path)
          n137 = Concatenate Strings(w194, w192, w207, w192, w206, w192, w199, w192, w198, w192, w197, w192, w196, w192, w195, w192, w190, "\r\n") -> (w183:string)
          n138 = call-poly "IMAQ Write File 2"("Image Quality"=u32 1000, "File Path"=w188, "Image"=w189) -> ()  [unwired: 7 in, 2 out]
          n139 = Write to Text File(file (use dialog)=w185, text=w183, error in=w184) -> (refnum out=w182:refnum<file>, error out=w181:errorcluster)  [unwired: 1 in, 1 out]
        }
        n140 = Close File(refnum=w173, error in=w172) -> ()  [unwired: 2 out]
      }
    }
    n141 = Increment(x=w14) -> (x+1=w11:i32)
    n142 = local write "currentImage"(w11) -> ()
  }
  "state" <- 0
  "Identified Targets" <- T2 [] ("Array")
